vi "read_TCUStatus3_2.vi"(1 "Array":u8[](array[numeric])=[0, 0, 0, 0, 0, 0, 0, 0, 0, 0, 0, 0, 0, 0, 0, 0, 0, 0, 0, 0, 0, 0, 0, 0, 0, 0, 0, 0, 0, 0, 0, 0, 0, 0, 0, 0, 0, 0, 0, 0, 0, 0, 0, 0, 0, 0, 0, 0, 0, 0, 0, 0, 0, 0, 0, 0, 0, 0, 0, 0, 0, 0, 0, 0, 0, 0, 0, 0, 0, 0, 0, 0, 0, 0, 0, 0, 0, 0, 0, 0, 0, 0, 0, 0, 0, 0, 0, 0, 0, 0, 0, 0, 0, 0, 0, 0, 0, 0, 0, 0, 0, 0, 0, 0, 0, 0, 0, 0, 0, 0, 0, 0, 0, 0, 0, 0, 0, 0, 0, 0, 0, 0, 0, 0, 0, 0, 0, 0, 0, 0, 0, 0, 0, 0, 0, 0, 0, 0, 0, 0, 0, 0, 0, 0, 0, 0, 0, 0, 0, 0, 0, 0, 0, 0, 0, 0, 0, 0, 0, 0, 0, 0, 0, 0, 0, 0, 0, 0, 0, 0, 0, 0, 0, 0, 0, 0, 0, 0, 0, 0, 0]) -> (0 "Message":T1)   [LabVIEW 2017]
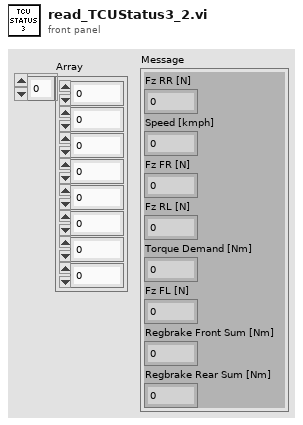
[diagram p1: front panel]
types:
  T1 = cluster{"Fz RR [N]":u16, "Speed [kmph]":dbl, "Fz FR [N]":u16, "Fz RL [N]":u16, "Torque Demand [Nm]":dbl, "Fz FL [N]":u16, "Regbrake Front Sum [Nm]":dbl, "Regbrake Rear Sum [Nm]":dbl}
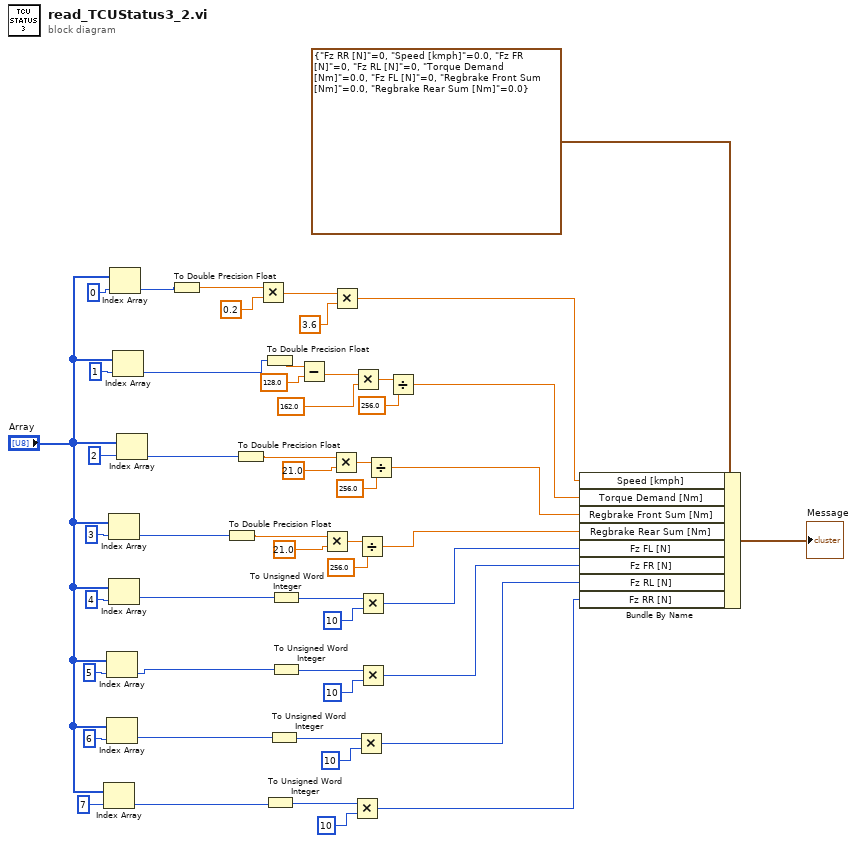
[diagram p0: block diagram]
diagram:
  n1 = Index Array(array="Array", index=7) -> (element=w5:u8)
  n2 = Index Array(array="Array", index=5) -> (element=w7:u8)
  n3 = Index Array(array="Array", index=6) -> (element=w6:u8)
  n4 = Index Array(array="Array", index=3) -> (element=w16:u8)
  n5 = Index Array(array="Array", index=4) -> (element=w40:u8)
  n6 = Index Array(array="Array", index=0) -> (element=w37:u8)
  n7 = Index Array(array="Array", index=1) -> (element=w30:u8)
  n8 = Index Array(array="Array", index=2) -> (element=w22:u8)
  n9 = To Double Precision Float(number=w37) -> (double precision float=w39:dbl)
  n10 = To Double Precision Float(number=w16) -> (double precision float=w20:dbl)
  n11 = To Double Precision Float(number=w22) -> (double precision float=w23:dbl)
  n12 = Multiply(x=w39, y=0.2) -> (x*y=w36:dbl)
  n13 = To Double Precision Float(number=w30) -> (double precision float=w34:dbl)
  n14 = To Unsigned Word Integer(number=w5) -> (unsigned 16bit integer=w9:u16)
  n15 = To Unsigned Word Integer(number=w6) -> (unsigned 16bit integer=w10:u16)
  n16 = To Unsigned Word Integer(number=w40) -> (unsigned 16bit integer=w41:u16)
  n17 = To Unsigned Word Integer(number=w7) -> (unsigned 16bit integer=w13:u16)
  n18 = Subtract(x=w34, y=128.0) -> (x-y=w32:dbl)
  n19 = Multiply(x=w20, y=21.0) -> (x*y=w18:dbl)
  n20 = Multiply(x=w23, y=21.0) -> (x*y=w25:dbl)
  n21 = Multiply(x=w36, y=3.6) -> (x*y=w43:dbl)
  n22 = Multiply(x=w9, y=u16 10) -> (x*y=w2:u16)
  n23 = Multiply(x=w32, y=162.0) -> (x*y=w29:dbl)
  n24 = Multiply(x=w10, y=u16 10) -> (x*y=w3:u16)
  n25 = Divide(x=w18, y=256.0) -> (x/y=w15:dbl)
  n26 = Multiply(x=w41, y=u16 10) -> (x*y=w14:u16)
  n27 = Multiply(x=w13, y=u16 10) -> (x*y=w4:u16)
  n28 = Divide(x=w25, y=256.0) -> (x/y=w21:dbl)
  n29 = Divide(x=w29, y=256.0) -> (x/y=w27:dbl)
  n30 = Bundle By Name(cluster=T1 {"Fz RR [N]"=0, "Speed [kmph]"=0.0, "Fz FR [N]"=0, "Fz RL [N]"=0, "Torque Demand [Nm]"=0.0, "Fz FL [N]"=0, "Regbrake Front Sum [Nm]"=0.0, "Regbrake Rear Sum [Nm]"=0.0}, "Speed [kmph]"=w43, "Torque Demand [Nm]"=w27, "Regbrake Front Sum [Nm]"=w21, "Regbrake Rear Sum [Nm]"=w15, "Fz FL [N]"=w14, "Fz FR [N]"=w4, "Fz RL [N]"=w3, "Fz RR [N]"=w2) -> (→"Message":T1)
